vi "toml_loads.vi"(8 "error in (no error)":errorcluster, 11 "path in":path) -> (0 "error out":errorcluster, 2 "file":T1, 3 "path out":path)   [LabVIEW 2017]
uses:
  toml_fg_file.ctl
  toml_fg_section.ctl
  toml_fg_row.ctl
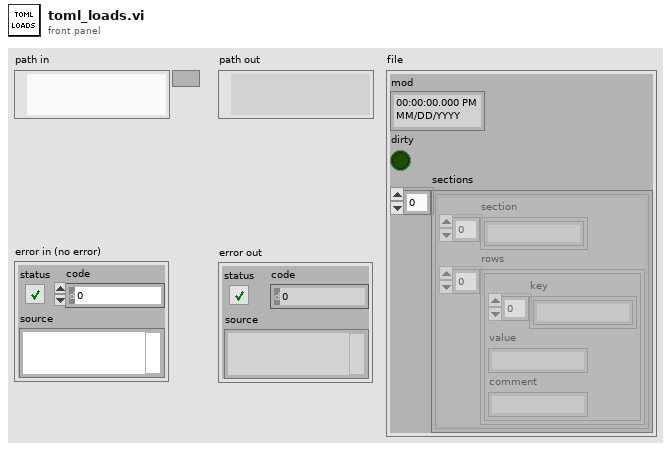
[diagram p1: front panel]
types:
  T1 = typedef "toml_fg_file.ctl" = cluster{"mod":timestamp, "dirty":bool, "sections":T2[]}
  T2 = typedef "toml_fg_section.ctl" = cluster{"section":string[], "rows":T3[]}
  T3 = typedef "toml_fg_row.ctl" = cluster{"key":string[], "value":string, "comment":string}
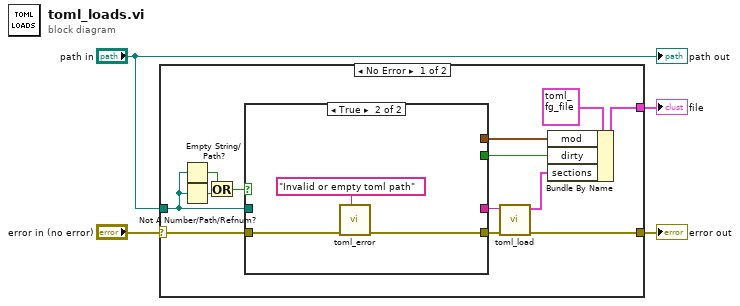
[diagram p0: block diagram]
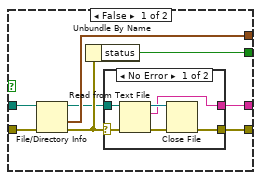
[diagram p2: hidden frame]
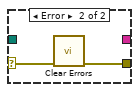
[diagram p3: hidden frame]
diagram:
  n1 = case shown="No Error" "error in (no error)" {
    selector: "error in (no error)" -> [w14 w37]
    tunnel: "path in" -> [w8 _]
    tunnel: [w11 w37] -> w2
    tunnel: [w10 _] -> w1
    frame No Error {
      n2 = Empty String/Path?(string/path=w8) -> (empty?=w6:bool)
      n3 = Not A Number/Path/Refnum?(number/path/refnum=w8) -> (NaN/Path/Refnum?=w7:bool)
      n4 = Or(x=w6, y=w7) -> (x .or. y?=w5:bool)
      n5 = case shown="True" w5 {
        tunnel: [w25 _] -> w16
        tunnel: [w24 _] -> w15
        tunnel: w14 -> [w23 w36]
        tunnel: [w20 w35] -> w13
        tunnel: [w19 _] -> w12
        tunnel: w8 -> [w18 _]
        frame False {
          n6 = File/Directory Info(path=w18, error in=w23) -> (path out=w21:path, last mod=w25:timestamp, error out=w22:errorcluster)  [unwired: 4 out]
          n7 = Unbundle By Name(w22) -> ("status"=w24:bool)
          n8 = case shown="No Error" w22 {
            selector: w22 -> [w29 w33]
            tunnel: w21 -> [w28 _]
            tunnel: [w27 w32] -> w20
            tunnel: [w26 _] -> w19
            frame No Error {
              n9 = Read from Text File(file (use dialog)=w28, error in=w29) -> (refnum out=w30:refnum<file>, text=w26:string, error out=w31:errorcluster)  [unwired: 2 in, 1 out]
              n10 = Close File(refnum=w30, error in=w31) -> (error out=w27:errorcluster)  [unwired: 1 out]
            }
            frame Error {
              n11 = call <vilib>:"Clear Errors.vi"("error in (no error)"=w33) -> ("error out"=w32:errorcluster)  [unwired: 5 in, 1 out]
            }
          }
        }
        frame True {
          n12 = call "toml_error.vi"("message"="Invalid or empty toml path", "error in (no error)"=w36) -> ("error out"=w35:errorcluster)  [unwired: 9 in]
        }
      }
      n13 = call "toml_load.vi"("error in (no error)"=w13, "toml"=w12) -> ("error out"=w11:errorcluster, "sections"=w9:T2[])  [unwired: 8 in]
      n14 = Bundle By Name(cluster=T1 {"mod"=timestamp(0 s since 1904-01-01), "dirty"=FALSE, "sections"=[]} ("file"), "mod"=w16, "dirty"=w15, "sections"=w9) -> (w10:T1)
    }
    frame Error {
    }
  }
  "error out" <- w2
  "file" <- w1
  "path out" <- "path in"
